vi "create backup files.vi"(8 "error in (no error)":errorcluster caption="错误输入（无错误）", 10 "execute file name":string, 11 "路径":path) -> (0 "error out":errorcluster caption="错误输出")   [LabVIEW 2016, in "数据传输系统-04.lvlib" / "update.lvlib"]
uses:
  update.lvlib
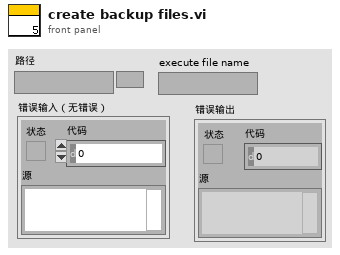
[diagram p1: front panel]
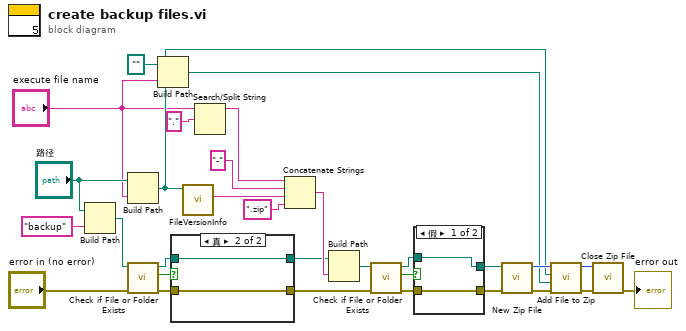
[diagram p0: block diagram]
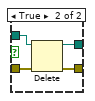
[diagram p2: hidden frame]
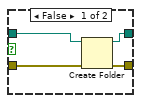
[diagram p3: hidden frame]
diagram:
  n1 = Build Path(base path="路径", name or relative path="backup" ("名称或相对路径")) -> (appended path=w17:path)
  n2 = Build Path(base path="路径", name or relative path="execute file name") -> (appended path=w2:path)
  n3 = call <vilib>:"Check if File or Folder Exists.vi"("error in (no error)"="error in (no error)", "path"=w17) -> ("error out"=w7:errorcluster, "file or folder exists?"=w16:bool, "dup path"=w15:path)  [unwired: 7 in]
  n4 = Build Path(base path=path "" ("Relative Path from 1 to 2"), name or relative path="execute file name") -> (appended path=w18:path)
  n5 = case shown="真" w16 {
    tunnel: w15 -> [w34 w36]
    tunnel: [w33 w36] -> w14
    tunnel: w7 -> [w32 w35]
    tunnel: [w31 w35] -> w6
    frame False {
      n6 = Create Folder(path (use dialog)=w34, error in=w32) -> (created path=w33:path, error out=w31:errorcluster)  [unwired: 1 in, 1 out]
    }
    frame True {
    }
  }
  n7 = call <vilib>:"FileVersionInfo.vi"("Application Path in"=w2) -> ("File Version Info"=w28:string)  [unwired: 7 in, 3 out]
  n8 = Search/Split String(string="execute file name", search string/char (-)="." ("搜索字符串/字符(-)")) -> (substring before match=w25:string)  [unwired: 1 in, 2 out]
  n9 = Concatenate Strings(w25, "-" ("字符串"), w28, ".zip" ("字符串")) -> (w24:string)
  n10 = Build Path(base path=w14, name or relative path=w24) -> (appended path=w11:path)
  n11 = call <vilib>:"Check if File or Folder Exists.vi"("error in (no error)"=w6, "path"=w11) -> ("error out"=w9:errorcluster, "file or folder exists?"=w12:bool, "dup path"=w13:path)  [unwired: 7 in]
  n12 = case shown="假" w12 {
    tunnel: w13 -> [w38 w42]
    tunnel: [w38 w41] -> w10
    tunnel: w9 -> [w37 w40]
    tunnel: [w37 w39] -> w8
    frame False {
    }
    frame True {
      n13 = Delete(path (use dialog)=w42, error in=w40) -> (deleted path=w41:path, error out=w39:errorcluster)  [unwired: 3 in, 1 out]
    }
  }
  n14 = call <vilib>:"New Zip File.vi"("error in (no error)"=w8, "target"=w10) -> ("error out"=w23:errorcluster, "zip file out"=w22:i64)  [unwired: 1 in, 3 out]
  n15 = call <vilib>:"Add File to Zip.vi"("error in (no error)"=w23, "destination path in zip"=w18, "source file path"=w2, "zip file in"=w22) -> ("error out"=w20:errorcluster, "zip file out"=w21:i64)  [unwired: 6 in]
  n16 = call <vilib>:"Close Zip File.vi"("error in (no error)"=w20, "zip file in"=w21) -> ("error out"=→"error out":errorcluster)  [unwired: 5 in]
